vi "WPI_CANTalonSRX_MotionProfile_TrajGlobal.vi"(8 "Trajectory Point To Store":T1, 9 "Is Store":bool, 11 "Device ID (0)":u8) -> (0 "Read For Send":T1, 3 "Device ID Out":u8)   [LabVIEW 2016]
uses:
  <vilib>/Rock Robotics/WPI/ThirdParty/CanMotor/TalonSRX/WPI_CANTalonSRX_MotionProfileTrajectoryPt.ctl
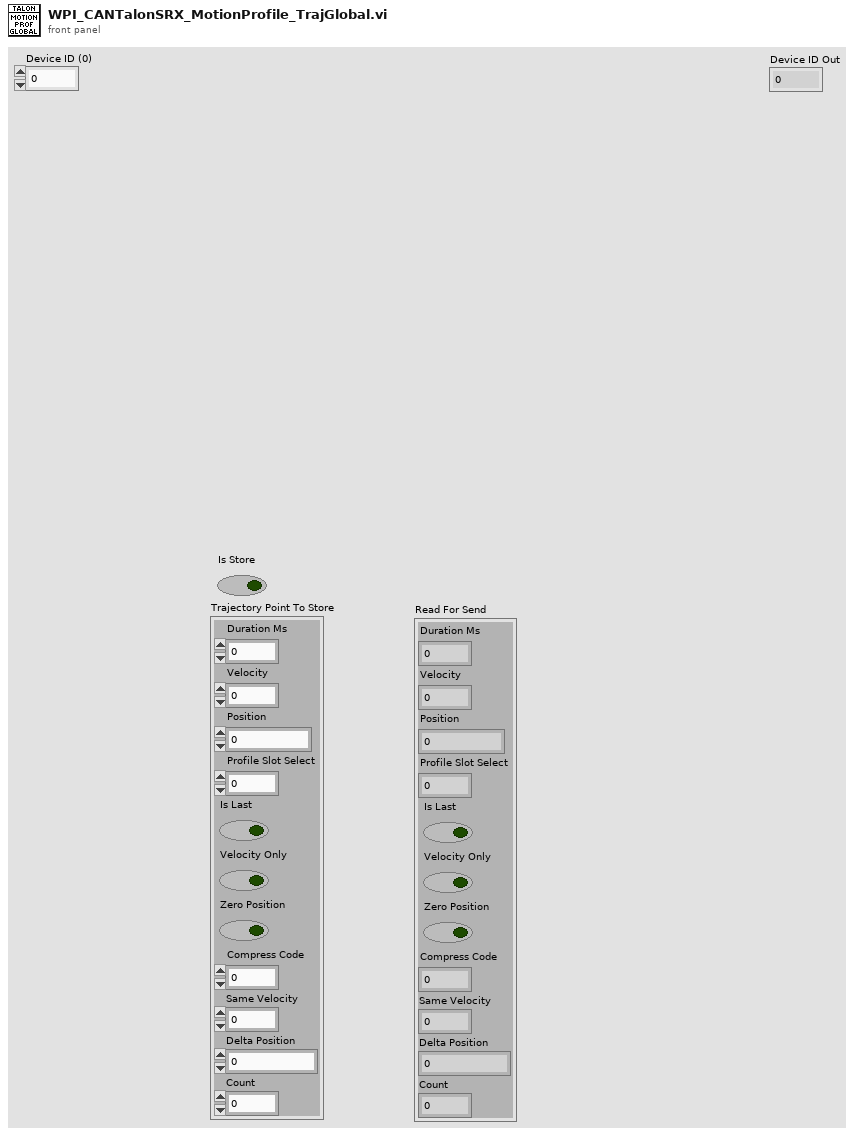
[diagram p1: front panel]
types:
  T1 = typedef "WPI_CANTalonSRX_MotionProfileTrajectoryPt.ctl" = cluster{"Duration Ms":u8, "Velocity":dbl, "Position":dbl, "Profile Slot Select":u8, "Is Last":bool, "Velocity Only":bool, "Zero Position":bool, "Compress Code":u8, "Same Velocity":i32, "Delta Position":i32, "Count":u8}
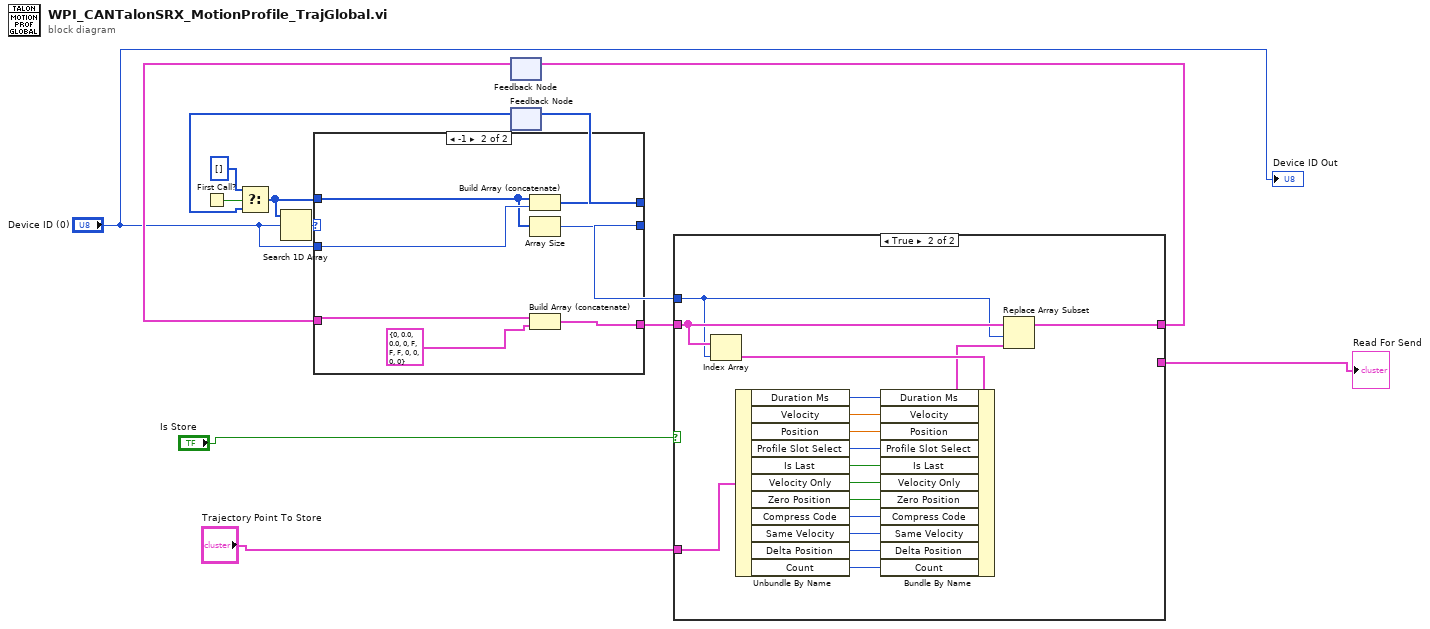
[diagram p0: block diagram]
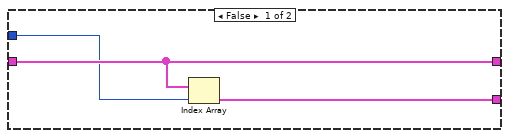
[diagram p2: hidden frame]
diagram:
  n1 = First Call?() -> (First Call?: T/F=w14:bool)
  n2 = feedback #1() -> (w8:T1[])  [unwired: 1 in]
  n3 = feedback #2() -> (w12:u8[])  [unwired: 1 in]
  n4 = Select(t=u8[] [], s=w14, f=w12) -> (s? t:f=w10:u8[])
  n5 = Search 1D Array(1D array=w10, element="Device ID (0)") -> (index of element=w9:i32)  [unwired: 1 in]
  n6 = case shown="-1" w9 {
    selector: w9 -> [w15 _]
    tunnel: [w17 w24] -> w11
    tunnel: "Device ID (0)" -> [_ w23]
    tunnel: w10 -> [w17 w20]
    tunnel: w8 -> [w16 w22]
    tunnel: [w16 w21] -> w6
    tunnel: [w15 w19] -> w5
    frame Default {
    }
    frame -1 {
      n7 = Build Array (concatenate)(w20, w23) -> (w24:u8[])
      n8 = Array Size(array=w20) -> (size(s)=w19:i32)
      n9 = Build Array (concatenate)(w22, T1 {"Duration Ms"=0, "Velocity"=0.0, "Position"=0.0, "Profile Slot Select"=0, "Is Last"=FALSE, "Velocity Only"=FALSE, "Zero Position"=FALSE, "Compress Code"=0, "Same Velocity"=0, "Delta Position"=0, "Count"=0} ("Talon SRX Motion Profile Trajectory Point")) -> (w21:T1[])
    }
  }
  n10 = feedback-in #2(w11) -> ()
  n11 = case shown="True" "Is Store" {
    tunnel: [w27 w44] -> w7
    tunnel: w6 -> [w27 w43]
    tunnel: w5 -> [w26 w42]
    tunnel: [w25 _] -> w2
    tunnel: "Trajectory Point To Store" -> [_ w39]
    frame False {
      n12 = Index Array(array=w27, index=w26) -> (element=w25:T1)
    }
    frame True {
      n13 = Index Array(array=w43, index=w42) -> (element=w41:T1)
      n14 = Unbundle By Name(w39) -> ("Duration Ms"=w38:u8, "Velocity"=w37:dbl, "Position"=w36:dbl, "Profile Slot Select"=w35:u8, "Is Last"=w34:bool, "Velocity Only"=w33:bool, "Zero Position"=w32:bool, "Compress Code"=w31:u8, "Same Velocity"=w30:i32, "Delta Position"=w29:i32, "Count"=w28:u8)
      n15 = Bundle By Name(cluster=w41, "Duration Ms"=w38, "Velocity"=w37, "Position"=w36, "Profile Slot Select"=w35, "Is Last"=w34, "Velocity Only"=w33, "Zero Position"=w32, "Compress Code"=w31, "Same Velocity"=w30, "Delta Position"=w29, "Count"=w28) -> (w40:T1)
      n16 = Replace Array Subset(array=w43, new element=w40, index=w42) -> (w44:T1[])
    }
  }
  "Read For Send" <- w2
  n17 = feedback-in #1(w7) -> ()
  "Device ID Out" <- "Device ID (0)"
